vi "Run Action.vi"(6 "Timeout (s)":dbl, 8 "ErrorIn":errorcluster, 9 "IAction":refnum<class "IAction.lvclass">, 10 "Action":string, 11 "TopModuleIn":refnum<class "TopModule.lvclass">) -> (0 "ErrorOut":errorcluster, 1 "Timeout?":bool, 3 "TopModuleOut":refnum<class "TopModule.lvclass">)   [LabVIEW 2020, in "TopModule.lvclass"]
uses:
  TopModule.lvclass
  TopModule.lvclass/TopModule.ctl
  IAction/IAction.lvclass
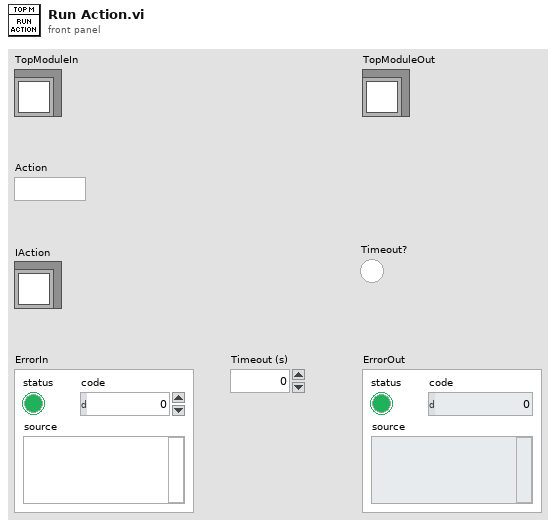
[diagram p1: front panel]
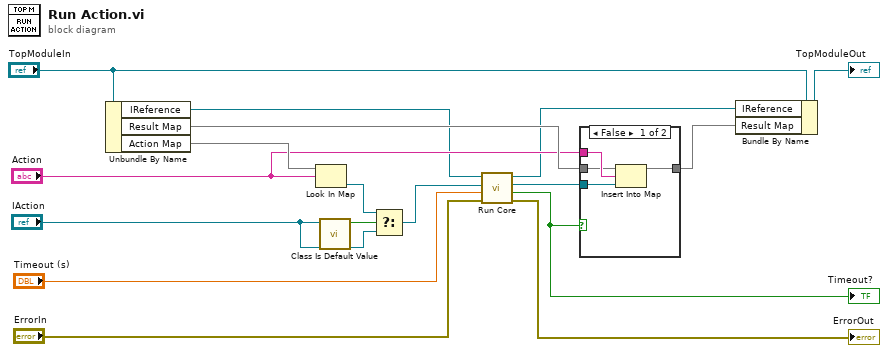
[diagram p0: block diagram]
diagram:
  n1 = Unbundle By Name("TopModuleIn") -> ("IReference"=w11:refnum<class "IRef.lvclass">, "Result Map"=w14:map{string, refnum<class "IResult.lvclass">}, "Action Map"=w15:map{string, refnum<class "IAction.lvclass">})
  n2 = Look In Map(map=w15, key="Action") -> (value=w4:refnum<class "IAction.lvclass">)  [unwired: 1 in, 1 out]
  n3 = call "Class Is Default Value.vi"("Object"="IAction") -> ("Default Value"=w2:bool)  [unwired: 10 in]
  n4 = Select(t=w4, s=w2, f="IAction") -> (s? t:f=w3:refnum<class "IAction.lvclass">)
  n5 = call-dynamic "Run Core.vi"("Error In"="ErrorIn", "Timeout (s)"="Timeout (s)", "IAction In"=w3, "Reference In"=w11) -> ("Error Out"=→"ErrorOut":errorcluster, "Timeout?"=w6:bool, "IResult Out"=w5:refnum<class "IResult.lvclass">, "Reference Out"=w10:refnum<class "IRef.lvclass">)  [unwired: 4 in]
  "Timeout?" <- w6
  n6 = case shown="False" w6 {
    tunnel: "Action" -> [w21 _]
    tunnel: w14 -> [w20 w22]
    tunnel: [w19 w22] -> w13
    tunnel: w5 -> [w18 _]
    frame False {
      n7 = Insert Into Map(map in=w20, key=w21, value=w18) -> (map out=w19:map{string, refnum<class "IResult.lvclass">})  [unwired: 2 out]
    }
    frame True {
    }
  }
  n8 = Bundle By Name(cluster="TopModuleIn", "IReference"=w10, "Result Map"=w13) -> (→"TopModuleOut":refnum<class "TopModule.lvclass">)
